vi "PP.ReadFile.To.ByteArray.vi"(8 "error in":errorcluster, 11 "file path (use dialog)":path) -> (0 "error out":errorcluster, 2 "data":u8[](array[numeric]), 3 "file path out":path)   [LabVIEW 2020, in "PixPack.lvlib"]
uses:
  PixPack.lvlib
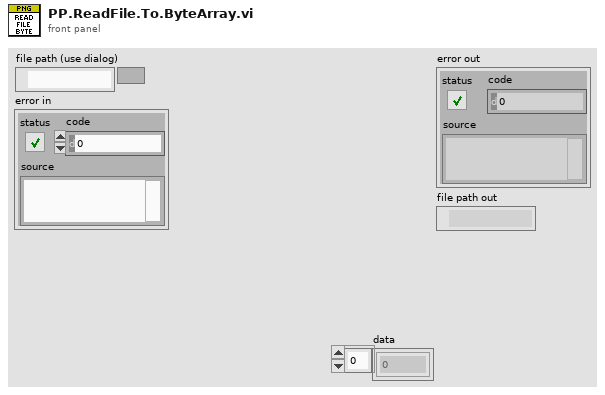
[diagram p1: front panel]
types:
  T1 = enum16{"big-endian, network order", "native, host order", "little-endian"}
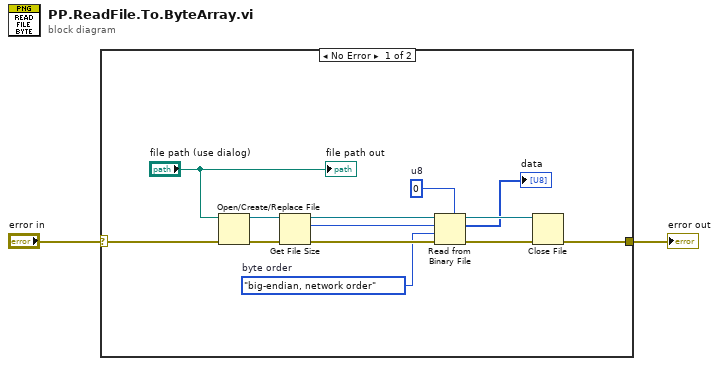
[diagram p0: block diagram]
diagram:
  n1 = case shown="No Error" "error in" {
    selector: "error in" -> [w6 w16]
    tunnel: [w4 w16] -> w1
    frame No Error {
      w7 = T1."big-endian, network order"  # byte order
      w8 = u8 0  # u8
      n2 = Open/Create/Replace File(file path (use dialog)="file path (use dialog)", error in=w6) -> (refnum out=w9:refnum<file>, error out=w12:errorcluster)  [unwired: 4 in, 1 out]
      n3 = Get File Size(file=w9, error in=w12) -> (refnum out=w10:refnum<file>, size (in bytes)=w11:i64, 0:w13:errorcluster)
      n4 = Read from Binary File(5:w8, 8:w13, 9:w7, 10:w11, 11:w10) -> (0:w14:errorcluster, 2:→"data":u8[], 3:w15:refnum<file>)  [unwired: 1 in, 1 out]
      n5 = Close File(refnum=w15, error in=w14) -> (error out=w4:errorcluster)  [unwired: 1 out]
      "file path out" <- "file path (use dialog)"
    }
    frame Error {
    }
  }
  "error out" <- w1
